vi "lane_test1.vi"(11 "lane_body":dbl[][](array[numeric])) -> ()   [LabVIEW 2015]
uses:
  G_VEH.vi
  G_NAV.vi
  G_PATH.vi
panel:
  out "Array":i32[](array[numeric])
  out "cross":dbl[][](array[numeric])
  out "seed":dbl[](array[numeric])
  out "seedr1":dbl=-1.5
  out "lane":dbl[][](array[numeric])
  out "path":dbl[](array[numeric])
  out "error out 2":errorcluster caption="error out"
  out "x_path":dbl[](array[numeric])
  out "y_path":dbl[](array[numeric])
  out "x_path2":dbl[](array[numeric])
  out "XY Graph":cluster{"Y":dbl[], "Y":dbl[]}[](graph)
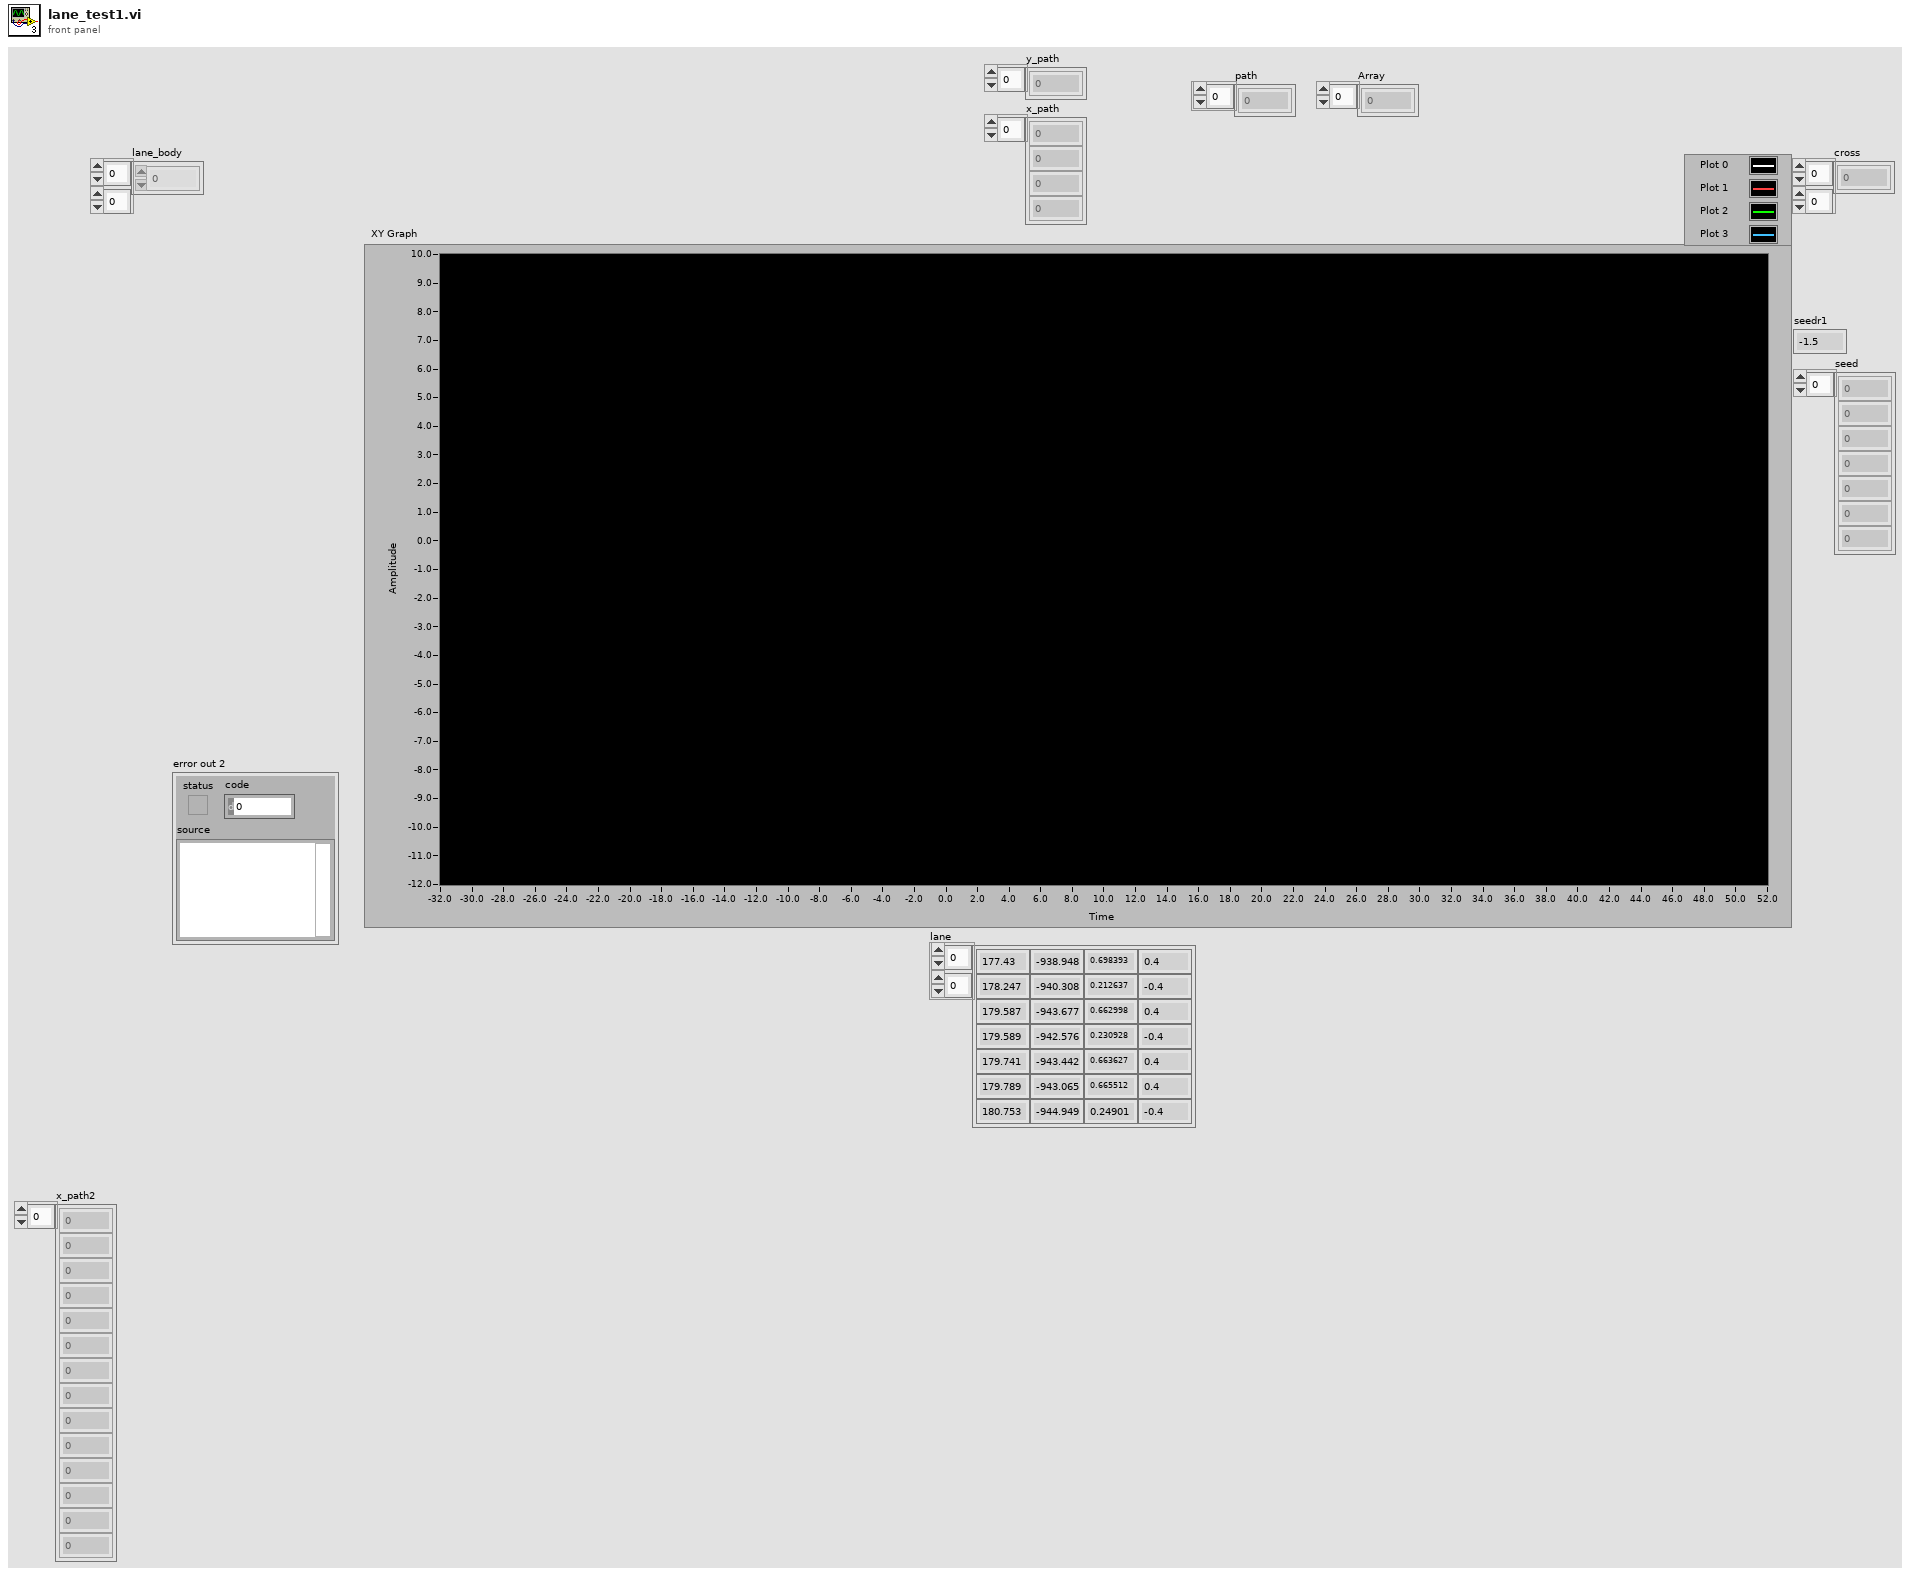
[diagram p1: front panel]
types:
  T1 = cluster{"Steer_input":dbl, "Steer_output":dbl, "VS_des":dbl, "VS_can":dbl, "heading":dbl, "auto":bool, "run":bool, "x":dbl, "y":dbl}
  T2 = cluster{"idx":i32, "x":dbl, "y":dbl, "h":dbl, "x_path":dbl}
  T3 = cluster{"GPSTime":dbl, "attitude[2]":dbl, "lcc[0]":dbl, "lcc[1]":dbl, "heading_GPS":dbl}
  T4 = cluster{"element":i16, "element":dbl, "element":dbl}[]
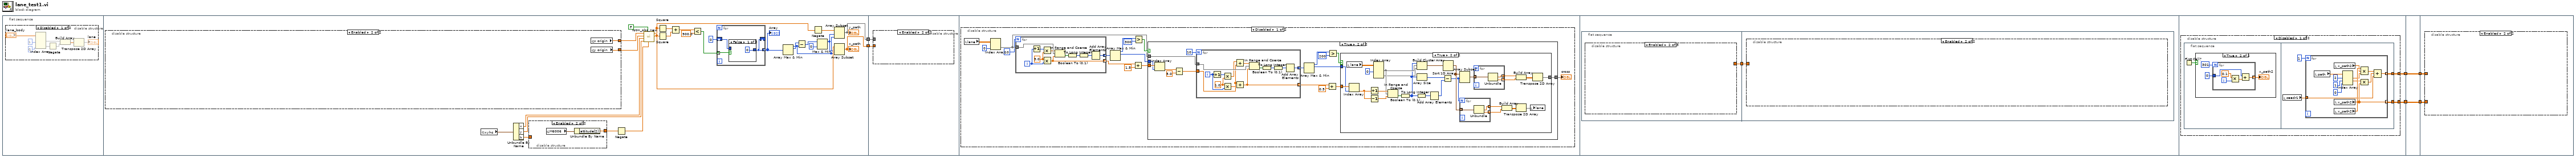
[diagram p0: block diagram]
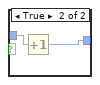
[diagram p3: hidden frame]
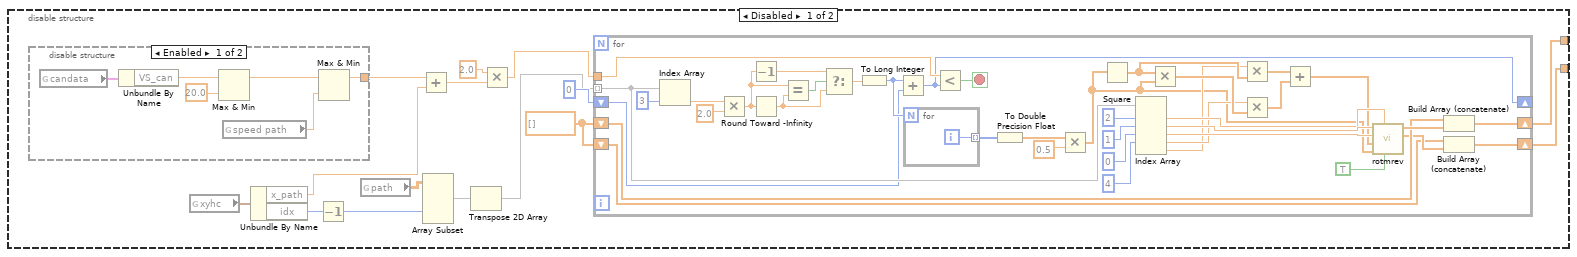
[diagram p4: hidden frame]
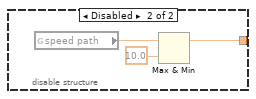
[diagram p5: hidden frame]
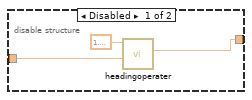
[diagram p6: hidden frame]
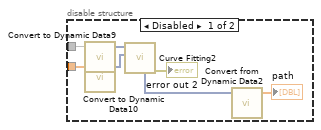
[diagram p7: hidden frame]
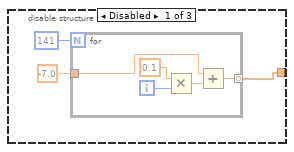
[diagram p11: hidden frame]
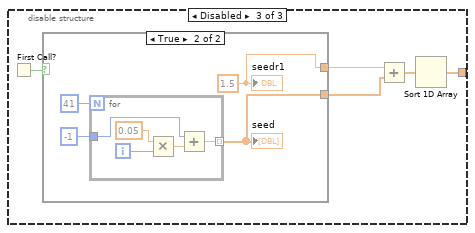
[diagram p12: hidden frame]
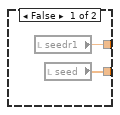
[diagram p13: hidden frame]
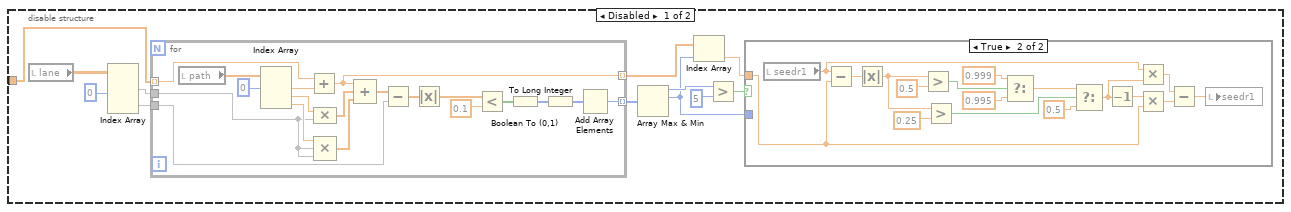
[diagram p14: hidden frame]
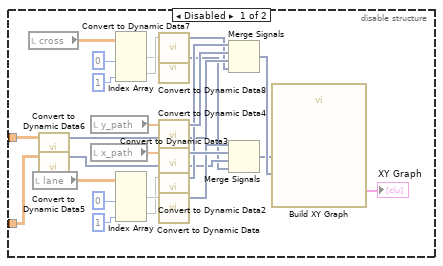
[diagram p18: hidden frame]
diagram:
  n1 = flat-sequence {
    tunnel: [w30] -> w2
    tunnel: [w29] -> w1
    tunnel: w2 -> [w119]
    tunnel: w1 -> [w118]
    tunnel: [w287] -> w5
    tunnel: [w286] -> w3
    tunnel: [w317] -> w6
    tunnel: w5 -> [w317]
    tunnel: [w316] -> w4
    tunnel: w3 -> [w316]
    tunnel: w6 -> [w319]
    tunnel: w4 -> [w318]
    frame #0 {
      n2 = disable-structure shown="Disabled" {
        frame Disabled {
          n3 = Index Array(array="lane_body", index (col) #1=1 ("disabled index (col)"), index (col) #2=0 ("index (col)")) -> (element #1=w12:dbl[], element #2=w13:dbl[])  [unwired: 2 in]
          n4 = Negate(x=w13) -> (-x=w11:dbl[])
          n5 = Build Array(w12, w11) -> (w10:dbl[][])
          n6 = Transpose 2D Array(2D array=w10) -> (transposed array=→"lane":dbl[][])
        }
        frame Enabled {
        }
      }
    }
    frame #1 {
      n7 = disable-structure shown="Enabled" {
        disable-tunnel: [w48 w112] -> w33
        disable-tunnel: [w47 w111] -> w32
        frame Disabled {
          w55 = dbl[] []
          n8 = disable-structure shown="Enabled" {
            disable-tunnel: [w62 w68] -> w61
            frame Enabled {
              n9 = global read "G_VEH.vi" "candata"() -> (w67:T1)
              n10 = Unbundle By Name(w67) -> ("VS_can"=w66:dbl)
              n11 = Max & Min(x=w66, y=20.0) -> (max(x,y)=w64:dbl)  [unwired: 1 out]
              n12 = global read "G_VEH.vi" "speed path"() -> (w63:dbl)
              n13 = Max & Min(x=w64, y=w63) -> (max(x,y)=w62:dbl)  [unwired: 1 out]
            }
            frame Disabled {
              n14 = global read "G_VEH.vi" "speed path"() -> (w70:dbl)
              n15 = Max & Min(x=w70, y=10.0) -> (max(x,y)=w68:dbl)  [unwired: 1 out]
            }
          }
          n16 = global read "G_VEH.vi" "xyhc"() -> (w49:T2)
          n17 = Unbundle By Name(w49) -> ("x_path"=w60:dbl, "idx"=w50:i32)
          n18 = Decrement(x=w50) -> (x-1=w51:i32)
          n19 = global read "G_PATH.vi" "path"() -> (w52:dbl[][])
          n20 = Add(x=w61, y=w60) -> (x+y=w56:dbl)
          n21 = Array Subset(array=w52, index (col)=w51) -> (w53:dbl[][])  [unwired: 3 in]
          n22 = Transpose 2D Array(2D array=w53) -> (transposed array=w54:dbl[][])
          n23 = Multiply(x=2.0, y=w56) -> (x*y=w58:dbl)
          n24 = for {
            tunnel: w54 -> [w83] mode=indexing
            shift-right: [w80] -> w48
            shift-left: w55 -> [w79]
            shift-right: [w77] -> w47
            shift-left: w55 -> [w76]
            tunnel: w58 -> [w73]
            shift-right: [w72] -> _
            shift-left: 0 -> [w74]
            stop <- w71 stop-if-true
            n25 = Index Array(array=w83, index=3) -> (element=w108:dbl)
            n26 = Multiply(x=w108, y=2.0) -> (x*y=w106:dbl)
            n27 = Decrement(x=w106) -> (x-1=w104:dbl)
            n28 = Round Toward -Infinity(1:w106) -> (0:w103:dbl)
            n29 = Equal?(x=w106, y=w103) -> (x = y?=w105:bool)
            n30 = Select(t=w104, s=w105, f=w103) -> (s? t:f=w102:dbl)
            n31 = To Long Integer(number=w102) -> (32bit integer=w75:i32)
            n32 = Add(x=w75, y=w74) -> (x+y=w72:i32)
            n33 = for {
              N: w75 -> [_]
              tunnel: [w110] -> w101 mode=indexing
              i -> [w110]
            }
            n34 = Less?(x=w73, y=w72) -> (x < y?=w71:bool)
            n35 = To Double Precision Float(number=w101) -> (double precision float=w100:dbl[])
            n36 = Multiply(x=w100, y=0.5) -> (x*y=w82:dbl[])
            n37 = Square(x=w82) -> (x^2=w86:dbl[])
            n38 = Index Array(array=w83, index #1=2 ("index"), index #2=1 ("index"), index #3=0 ("index"), index #4=4 ("index")) -> (element #1=w95:dbl, element #2=w96:dbl, element #3=w97:dbl, element #4=w87:dbl, element #5=w85:dbl)  [unwired: 1 in]
            n39 = Multiply(x=w86, y=w82) -> (x*y=w88:dbl[])
            n40 = Multiply(x=w85, y=w86) -> (x*y=w89:dbl[])
            n41 = Multiply(x=w87, y=w88) -> (x*y=w90:dbl[])
            n42 = Add(x=w89, y=w90) -> (x+y=w91:dbl[])
            n43 = call "rotmrev.vi"("reverse"=TRUE, "angle[rad]"=w95, "x"=w82, "y"=w91, "x0"=w97, "y0"=w96) -> ("y"=w78:dbl[], "x"=w81:dbl[])  [unwired: 4 in]
            n44 = Build Array (concatenate)(w79, w81) -> (w80:dbl[])
            n45 = Build Array (concatenate)(w76, w78) -> (w77:dbl[])
          }
        }
        frame Enabled {
          n46 = global read "G_PATH.vi" "x origin"() -> (w112:dbl[])
          n47 = global read "G_PATH.vi" "y origin"() -> (w111:dbl[])
        }
      }
      n48 = global read "G_VEH.vi" "xyhc"() -> (w35:T2)
      n49 = Unbundle By Name(w35) -> ("x"=w36:dbl, "y"=w37:dbl, "h"=w38:dbl)
      n50 = disable-structure shown="Enabled" {
        disable-tunnel: w38 -> [w114 _]
        disable-tunnel: [w113 w116] -> w40
        frame Disabled {
          n51 = call "headingoperater.vi"("h1"=w114, "h2"=1.5707963267948966) -> ("h2-h1"=w113:dbl)  [unwired: 8 in, 1 out]
        }
        frame Enabled {
          n52 = global read "G_NAV.vi" "M6006"() -> (w117:T3)
          n53 = Unbundle By Name(w117) -> ("attitude[2]"=w116:dbl)
        }
      }
      n54 = Negate(x=w40) -> (-x=w39:dbl)
      n55 = call "rotm_obs_new.vi"("angle[rad]"=w39, "reverse"=FALSE, "y0"=w37, "x0"=w36, "y"=w32, "x"=w33) -> ("rot*(y-y0) 2"=w27:dbl[], "rot*(x-x0)"=w28:dbl[])  [unwired: 2 in, 2 out]
      n56 = Square(x=w28) -> (x^2=w26:dbl[])
      n57 = Square(x=w27) -> (x^2=w25:dbl[])
      n58 = Add(x=w26, y=w25) -> (x+y=w24:dbl[])
      n59 = Less?(x=w24, y=900.0) -> (x < y?=w22:bool[])
      n60 = for {
        tunnel: w22 -> [w43] mode=indexing
        shift-right: [w41] -> _
        shift-left: 0 -> [w42]
        tunnel: [w41] -> w20 mode=indexing
        n61 = case shown="False" w43 {
          tunnel: w42 -> [_ w46]
          tunnel: [0 w45] -> w41
          frame False {
          }
          frame True {
            n62 = Increment(x=w46) -> (x+1=w45:i32)
          }
        }
      }
      "Array" <- w20
      n63 = Array Max & Min(array=w20) -> (max value=w15:i32, max index (indices)=w19:i32)  [unwired: 2 out]
      n64 = Subtract(x=w19, y=w15) -> (x-y=w18:i32)
      n65 = Negate(x=w28) -> (-x=w31:dbl[])
      n66 = Max & Min(x=w18, y=0) -> (max(x,y)=w16:i32)  [unwired: 1 out]
      n67 = Array Subset(array=w31, index=w16, length=w15) -> (w30:dbl[])
      "y_path" <- w30
      n68 = Array Subset(array=w27, index=w16, length=w15) -> (w29:dbl[])
      "x_path" <- w29
    }
    frame #2 {
      n69 = disable-structure shown="Enabled" {
        disable-tunnel: w119 -> [w121 _]
        disable-tunnel: w118 -> [w120 _]
        frame Disabled {
          n70 = call "Convert to Dynamic Data9"("Array"=w121) -> ("Dynamic Data Type"=w123:dynamicdata)  [unwired: 3 in]
          n71 = call "Convert to Dynamic Data10"("Array"=w120) -> ("Dynamic Data Type"=w124:dynamicdata)  [unwired: 3 in]
          n72 = call "Curve Fitting2"("Locations"=w124, "Signals"=w123) -> ("error out"=→"error out 2":errorcluster, "polynomial coefficients"=w125:dynamicdata)  [unwired: 5 in, 3 out]
          n73 = call "Convert from Dynamic Data2"("Dynamic Data Type"=w125) -> ("Array"=→"path":dbl[])  [unwired: 3 in]
        }
        frame Enabled {
        }
      }
    }
    frame #3 {
      n74 = disable-structure shown="Disabled" {
        frame Disabled {
          n75 = local read "lane"() -> (w139:dbl[][])
          n76 = Index Array(array=w139, index (col)=0 ("disabled index (col)")) -> (element=w132:dbl[])  [unwired: 1 in]
          n77 = for {
            N: 10 -> [_]
            tunnel: w132 -> [w149]
            tunnel: [w141] -> w131 mode=indexing
            tunnel: [w140] -> w130 mode=indexing
            i -> [w147]
            w145 = 3.0 ("min")
            n78 = Increment(x=w147) -> (x+1=w148:i32)
            n79 = Multiply(x=w148, y=w145) -> (x*y=w146:dbl)
            n80 = Multiply(x=w145, y=w147) -> (x*y=w140:dbl)
            n81 = In Range and Coerce(upper limit=w146, x=w149, lower limit=w140) -> (In Range?=w144:bool[])  [unwired: 1 out]
            n82 = Boolean To (0,1)(Boolean=w144) -> (0, 1=w143:i16[])
            n83 = To Long Integer(number=w143) -> (32bit integer=w142:i32[])
            n84 = Add Array Elements(numeric array=w142) -> (sum=w141:i32)
          }
          n85 = Array Max & Min(array=w131) -> (max value=w137:i32, max index (indices)=w134:i32)  [unwired: 2 out]
          n86 = Add(x=w130, y=1.5) -> (x+y=w128:dbl[])
          n87 = Greater?(x=w137, y=300) -> (0:w135:bool)
          n88 = case shown="True" w135 {
            tunnel: w134 -> [_ w164]
            tunnel: w128 -> [_ w165]
            tunnel: w132 -> [_ w158]
            tunnel: [_ w159] -> w133
            frame False {
            }
            frame True {
              n89 = Index Array(array=w165, index=w164) -> (element=w155:dbl)
              n90 = Subtract(x=w155, y=5.0) -> (x-y=w153:dbl)
              n91 = for {
                N: 10 -> [_]
                tunnel: w158 -> [w178]
                tunnel: [w166] -> w151 mode=indexing
                tunnel: [w171] -> w157 mode=indexing
                tunnel: w153 -> [w168]
                i -> [w176]
                w175 = 1.0 ("min")
                n92 = Increment(x=w176) -> (x+1=w177:i32)
                n93 = Multiply(x=w177, y=w175) -> (x*y=w170:dbl)
                n94 = Multiply(x=w175, y=w176) -> (x*y=w167:dbl)
                n95 = Add(x=w170, y=w168) -> (x+y=w169:dbl)
                n96 = Add(x=w168, y=w167) -> (x+y=w166:dbl)
                n97 = In Range and Coerce(upper limit=w169, x=w178, lower limit=w166) -> (In Range?=w174:bool[])  [unwired: 1 out]
                n98 = Boolean To (0,1)(Boolean=w174) -> (0, 1=w173:i16[])
                n99 = To Long Integer(number=w173) -> (32bit integer=w172:i32[])
                n100 = Add Array Elements(numeric array=w172) -> (sum=w171:i32)
              }
              n101 = Array Max & Min(array=w157) -> (max value=w163:i32, max index (indices)=w160:i32)  [unwired: 2 out]
              n102 = Add(x=w151, y=0.5) -> (x+y=w150:dbl[])
              n103 = Greater?(x=w163, y=200) -> (0:w162:bool)
              n104 = case shown="True" w162 {
                tunnel: w150 -> [_ w204]
                tunnel: w160 -> [_ w201]
                tunnel: [_ w179] -> w159
                frame False {
                }
                frame True {
                  n105 = local read "lane"() -> (w203:dbl[][])
                  n106 = Index Array(array=w204, index=w201) -> (element=w199:dbl)
                  n107 = Increment(x=w199) -> (x+1=w200:dbl)
                  n108 = Decrement(x=w199) -> (x-1=w198:dbl)
                  n109 = Index Array(array=w203, index (col) #1=0 ("disabled index (col)")) -> (element #1=w197:dbl[], element #2=w196:dbl[])  [unwired: 3 in]
                  n110 = In Range and Coerce(upper limit=w200, x=w197, lower limit=w198) -> (In Range?=w194:bool[])  [unwired: 1 out]
                  n111 = Boolean To (0,1)(Boolean=w194) -> (0, 1=w192:i16[])
                  n112 = To Long Integer(number=w192) -> (32bit integer=w191:i32[])
                  n113 = Build Cluster Array(w192, w197, w196) -> (w195:T4)
                  n114 = Array Size(array=w192) -> (size(s)=w193:i32)
                  n115 = Add Array Elements(numeric array=w191) -> (sum=w190:i32)
                  n116 = Subtract(x=w193, y=w190) -> (x-y=w184:i32)
                  n117 = Sort 1D Array(array=w195) -> (sorted array=w185:T4)
                  n118 = Array Subset(array=w185, index=w184) -> (w183:T4)  [unwired: 1 in]
                  n119 = for {
                    N: w184 -> [_]
                    tunnel: w185 -> [w210] mode=indexing
                    tunnel: [w209] -> w189 mode=indexing
                    tunnel: [w208] -> w188 mode=indexing
                    n120 = Unbundle(w210) -> ("element"=w209:dbl, "element"=w208:dbl)  [unwired: 1 out]
                  }
                  n121 = for {
                    tunnel: w183 -> [w207] mode=indexing
                    tunnel: [w206] -> w181 mode=indexing
                    tunnel: [w205] -> w180 mode=indexing
                    n122 = Unbundle(w207) -> ("element"=w206:dbl, "element"=w205:dbl)  [unwired: 1 out]
                  }
                  n123 = Build Array(w189, w188) -> (w187:dbl[][])
                  n124 = Build Array(w181, w180) -> (w182:dbl[][])
                  n125 = Transpose 2D Array(2D array=w187) -> (transposed array=w186:dbl[][])
                  n126 = local write "lane"(w186) -> ()
                  n127 = Transpose 2D Array(2D array=w182) -> (transposed array=w179:dbl[][])
                }
              }
            }
          }
          "cross" <- w133
        }
        frame Enabled {
        }
      }
    }
    frame #4 {
      n128 = flat-sequence {
        tunnel: [w212] -> w211
        tunnel: w211 -> [w237]
        frame #0 {
          n129 = disable-structure shown="Enabled" {
            disable-tunnel: [w213 _ w224] -> w212
            frame Disabled {
              n130 = for {
                N: 141 -> [_]
                tunnel: -7.0 -> [w217]
                tunnel: [w216] -> w213 mode=indexing
                i -> [w220]
                n131 = Multiply(x=0.1, y=w220) -> (x*y=w218:dbl)
                n132 = Add(x=w217, y=w218) -> (x+y=w216:dbl)
              }
            }
            frame Enabled {
            }
            frame Disabled {
              n133 = First Call?() -> (First Call?: T/F=w223:bool)
              n134 = case shown="True" w223 {
                tunnel: [w227 w231] -> w222
                tunnel: [w226 w228] -> w221
                frame False {
                  n135 = local read "seedr1"() -> (w227:dbl)
                  n136 = local read "seed"() -> (w226:dbl[])
                }
                frame True {
                  w231 = 1.5
                  n137 = for {
                    N: 41 -> [_]
                    tunnel: -1 -> [w234]
                    tunnel: [w232] -> w228 mode=indexing
                    i -> [w236]
                    n138 = Multiply(x=0.05, y=w236) -> (x*y=w233:dbl)
                    n139 = Add(x=w234, y=w233) -> (x+y=w232:dbl)
                  }
                  "seed" <- w228
                  "seedr1" <- w231
                }
              }
              n140 = Add(x=w222, y=w221) -> (x+y=w225:dbl[])
              n141 = Sort 1D Array(array=w225) -> (sorted array=w224:dbl[])
            }
          }
        }
        frame #1 {
          n142 = disable-structure shown="Enabled" {
            disable-tunnel: w237 -> [w241 _]
            frame Disabled {
              n143 = local read "lane"() -> (w249:dbl[][])
              n144 = Index Array(array=w249, index (col) #1=0 ("disabled index (col)")) -> (element #1=w247:dbl[], element #2=w246:dbl[])  [unwired: 3 in]
              n145 = for {
                tunnel: w241 -> [w272] mode=indexing
                tunnel: w247 -> [w282]
                tunnel: w246 -> [w277]
                tunnel: [w270] -> w240 mode=indexing
                tunnel: [w269] -> w245 mode=indexing
                n146 = local read "path"() -> (w285:dbl[])
                n147 = Index Array(array=w285, index #1=0 ("index")) -> (element #1=w271:dbl, element #2=w281:dbl, element #3=w283:dbl)  [unwired: 2 in]
                n148 = Add(x=w272, y=w271) -> (x+y=w270:dbl)
                n149 = Compound Arithmetic op=MULTIPLY(w281, w282) -> (w279:dbl[])
                n150 = Compound Arithmetic op=MULTIPLY(w283, w282, w282) -> (w280:dbl[])
                n151 = Compound Arithmetic op=ADD(w270, w279, w280) -> (w278:dbl[])
                n152 = Subtract(x=w278, y=w277) -> (x-y=w276:dbl[])
                n153 = Absolute Value(x=w276) -> (abs(x)=w275:dbl[])
                n154 = Less?(x=w275, y=0.1) -> (x < y?=w273:bool[])
                n155 = Boolean To (0,1)(Boolean=w273) -> (0, 1=w268:i16[])
                n156 = To Long Integer(number=w268) -> (32bit integer=w267:i32[])
                n157 = Add Array Elements(numeric array=w267) -> (sum=w269:i32)
              }
              n158 = Array Max & Min(array=w245) -> (max value=w243:i32, max index (indices)=w239:i32)  [unwired: 2 out]
              n159 = Index Array(array=w240, index=w239) -> (element=w238:dbl)
              n160 = Greater?(x=w243, y=5) -> (0:w242:bool)
              n161 = case shown="True" w242 {
                tunnel: w239 -> [_ _]
                tunnel: w238 -> [_ w259]
                frame False {
                }
                frame True {
                  n162 = local read "seedr1"() -> (w262:dbl)
                  n163 = Subtract(x=w262, y=w259) -> (x-y=w266:dbl)
                  n164 = Absolute Value(x=w266) -> (abs(x)=w255:dbl)
                  n165 = Greater?(x=w255, y=0.5) -> (0:w253:bool)
                  n166 = Greater?(x=w255, y=0.25) -> (0:w264:bool)
                  n167 = Select(t=0.999, s=w253, f=0.995 ("t")) -> (s? t:f=w250:dbl)
                  n168 = Select(t=w250, s=w264, f=0.5) -> (s? t:f=w261:dbl)
                  n169 = Decrement(x=w261) -> (x-1=w260:dbl)
                  n170 = Multiply(x=w262, y=w261) -> (x*y=w257:dbl)
                  n171 = Multiply(x=w260, y=w259) -> (x*y=w258:dbl)
                  n172 = Subtract(x=w257, y=w258) -> (x-y=w256:dbl)
                  n173 = local write "seedr1"(w256) -> ()
                }
              }
            }
            frame Enabled {
            }
          }
        }
      }
    }
    frame #5 {
      n174 = disable-structure shown="Disabled" {
        disable-tunnel: [w289 _] -> w287
        disable-tunnel: [w288 _] -> w286
        frame Disabled {
          n175 = flat-sequence {
            tunnel: [w302] -> w288
            tunnel: [w300] -> w289
            frame #0 {
              n176 = First Call?() -> (First Call?: T/F=w290:bool)
              n177 = case shown="True" w290 {
                frame False {
                }
                frame True {
                  n178 = for {
                    N: 301 -> [_]
                    tunnel: 0 -> [w295]
                    tunnel: [w294] -> w291 mode=indexing
                    i -> [w298]
                    n179 = Multiply(x=0.1, y=w298) -> (x*y=w296:dbl)
                    n180 = Add(x=w295, y=w296) -> (x+y=w294:dbl)
                  }
                  "x_path2" <- w291
                }
              }
            }
            frame #1 {
              n181 = local read "seedr1"() -> (w301:dbl)
              n182 = for {
                N: 1 -> [_]
                tunnel: [w312] -> w302 mode=indexing
                tunnel: w301 -> [w303]
                tunnel: [w304] -> w300 mode=indexing
                n183 = local read "path"() -> (w305:dbl[])
                n184 = local read "x_path2"() -> (w310:dbl[])
                n185 = local read "x_path2"() -> (w304:dbl[])
                n186 = local read "x_path2"() -> (w311:dbl[])
                n187 = Index Array(array=w305, index #1=2 ("index"), index #2=1 ("index"), index #3=0 ("index")) -> (element #1=w309:dbl, element #2=w306:dbl)  [unwired: 1 out]
                n188 = Compound Arithmetic op=MULTIPLY(w311, w310, w309) -> (w308:dbl[])
                n189 = Compound Arithmetic op=MULTIPLY(w306, w304) -> (w307:dbl[])
                n190 = Compound Arithmetic op=ADD(w308, w307, w303) -> (w312:dbl[])
              }
            }
          }
        }
        frame Enabled {
        }
      }
    }
    frame #6 {
    }
    frame #7 {
      n191 = disable-structure shown="Enabled" {
        disable-tunnel: w319 -> [w332 _]
        disable-tunnel: w318 -> [w330 _]
        frame Disabled {
          n192 = local read "cross"() -> (w324:dbl[][])
          n193 = local read "lane"() -> (w328:dbl[][])
          n194 = call "Convert to Dynamic Data6"("2D Array"=w330) -> ("Dynamic Data Type"=w329:dynamicdata)  [unwired: 3 in]
          n195 = call "Convert to Dynamic Data5"("2D Array"=w332) -> ("Dynamic Data Type"=w331:dynamicdata)  [unwired: 3 in]
          n196 = local read "y_path"() -> (w344:dbl[])
          n197 = local read "x_path"() -> (w333:dbl[])
          n198 = Index Array(array=w324, index (col) #1=0 ("disabled index (col)"), index (col) #2=1 ("index (col)")) -> (element #1=w320:dbl[], element #2=w321:dbl[])  [unwired: 2 in]
          n199 = Index Array(array=w328, index (col) #1=0 ("disabled index (col)"), index (col) #2=1 ("index (col)")) -> (element #1=w336:dbl[], element #2=w327:dbl[])  [unwired: 2 in]
          n200 = call "Convert to Dynamic Data7"("Array"=w321) -> ("Dynamic Data Type"=w323:dynamicdata)  [unwired: 3 in]
          n201 = call "Convert to Dynamic Data8"("Array"=w320) -> ("Dynamic Data Type"=w322:dynamicdata)  [unwired: 3 in]
          n202 = call "Convert to Dynamic Data4"("Array"=w344) -> ("Dynamic Data Type"=w342:dynamicdata)  [unwired: 3 in]
          n203 = call "Convert to Dynamic Data3"("Array"=w333) -> ("Dynamic Data Type"=w340:dynamicdata)  [unwired: 3 in]
          n204 = call "Convert to Dynamic Data2"("Array"=w327) -> ("Dynamic Data Type"=w338:dynamicdata)  [unwired: 3 in]
          n205 = call "Convert to Dynamic Data"("Array"=w336) -> ("Dynamic Data Type"=w337:dynamicdata)  [unwired: 3 in]
          n206 = Merge Signals(w338, w342, w329, w323) -> (w341:dynamicdata)
          n207 = Merge Signals(w337, w340, w331, w322) -> (w339:dynamicdata)
          n208 = call "Build XY Graph"("Y Input"=w341, "X Input"=w339) -> ("XY Graph"=→"XY Graph":cluster{"Y":dbl[], "Y":dbl[]}[])  [unwired: 3 in, 6 out]
        }
        frame Enabled {
        }
      }
    }
  }
